vi "read TBM configuration.vi"(8 "error in":errorcluster, 11 "EthernetIP editor node in":refnum<class "EIP Tag API editor node.lvclass">) -> (0 "error out":errorcluster, 2 "TBM configuration out":refnum<class "TBM configuration.lvclass">, 3 "EthernetIP editor node out":refnum<class "EIP Tag API editor node.lvclass">)   [LabVIEW 2013, in "EIP Tag API editor node.lvclass"]
uses:
  EIP Tag API editor node.lvclass
  <vilib>/NI/Tag Bus Module Framework/root configuration/TBM configuration.lvclass
  EIP Tag API editor node.lvclass/EIP Tag API editor node.ctl
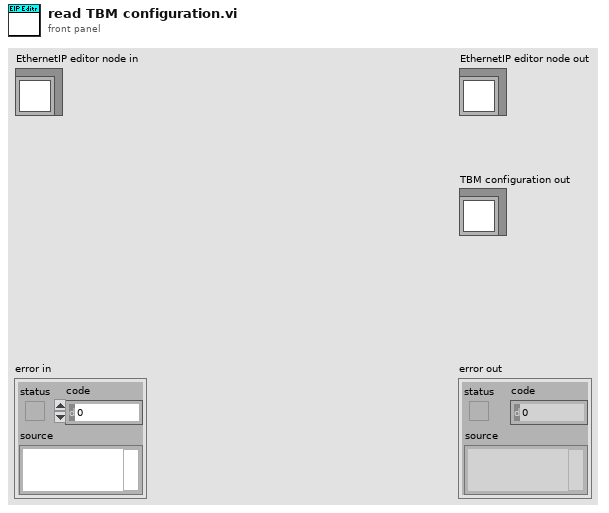
[diagram p1: front panel]
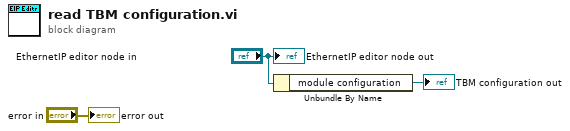
[diagram p0: block diagram]
diagram:
  n1 = Unbundle By Name("EthernetIP editor node in") -> ("module configuration"=→"TBM configuration out":refnum<class "EIP Tags Configuration.lvclass">)
  "error out" <- "error in"
  "EthernetIP editor node out" <- "EthernetIP editor node in"
